vi "Undo States.vi"(8 "error in":errorcluster, 10 "Expected Undo States":string[](array[string]), 11 "Test Case In":refnum<class "History Tests.lvclass">) -> (0 "error out":errorcluster, 2 "Actual Undo States":string[](array[string]), 3 "Test Case Out":refnum<class "History Tests.lvclass">)   [LabVIEW 2020, in "History Tests.lvclass"]
uses:
  History Tests.lvclass
  History Tests.lvclass/History Tests.ctl
  c447cda1-e09e-4100-8da7-89a8f417bcef.vi
  resource/plugins/NIIconEditor/History/History/History.lvclass
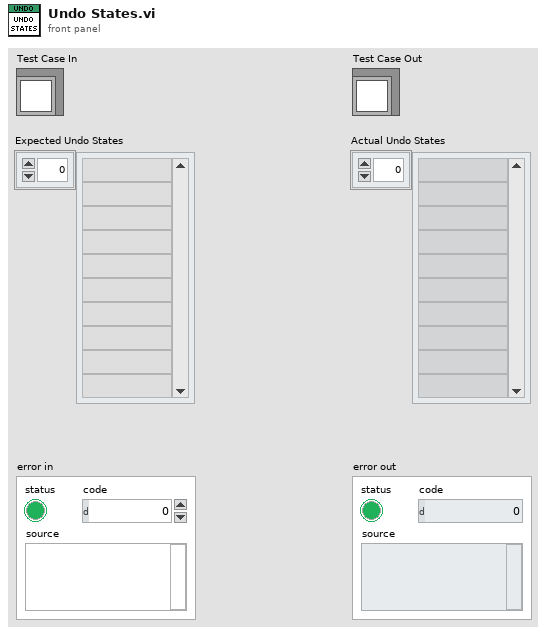
[diagram p1: front panel]
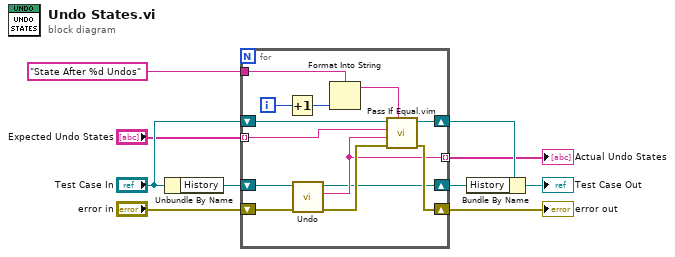
[diagram p0: block diagram]
diagram:
  n1 = Unbundle By Name("Test Case In") -> ("History"=w6:refnum<class "History.lvclass">)
  n2 = for {
    tunnel: [w13] -> w1 mode=indexing
    shift-right: [w18] -> w2
    shift-left: "Test Case In" -> [w19]
    tunnel: "Expected Undo States" -> [w20] mode=indexing
    shift-right: [w23] -> w9
    shift-left: "error in" -> [w22]
    tunnel: "State After %d Undos" ("Description") -> [w15]
    shift-right: [w11] -> w5
    shift-left: w6 -> [w12]
    i -> [w17]
    n3 = Increment(x=w17) -> (x+1=w14:i32)
    n4 = call "Undo.vi"("error in"=w22, "History in"=w12) -> ("error out"=w21:errorcluster, "State"=w13:string, "History out"=w11:refnum<class "History.lvclass">)  [unwired: 7 in]
    n5 = Format Into String(format string=w15, w14) -> (resulting string=w16:string)  [unwired: 2 in, 1 out]
    n6 = call "Pass If Equal.vim"("Description"=w16, "error in (no error)"=w21, "Actual"=w13, "Expected"=w20, "LUnit Test Case In"=w19) -> ("error out"=w23:errorcluster, "LUnit Test Case Out"=w18:refnum<class "History Tests.lvclass">)  [unwired: 5 in]
  }
  "error out" <- w9
  "Actual Undo States" <- w1
  n7 = Bundle By Name(cluster=w2, "History"=w5) -> (→"Test Case Out":refnum<class "History Tests.lvclass">)
